vi "archive items in folder.vi"() -> ()   [LabVIEW 2009]
panel:
  in  "suffixes to remove":string[](array[string])=[".vi  ", ".llb", ".txt "]
  out "Errors":errorcluster[](array[cluster])
  # "doesn't remove suffixes"
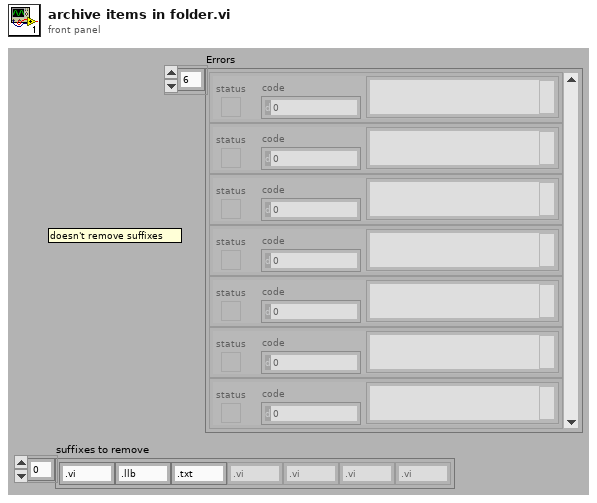
[diagram p1: front panel]
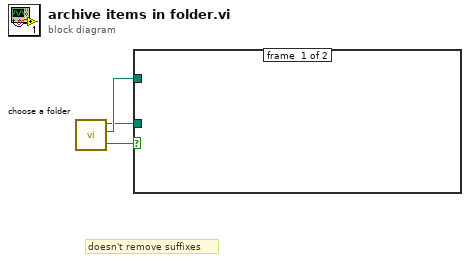
[diagram p0: block diagram]
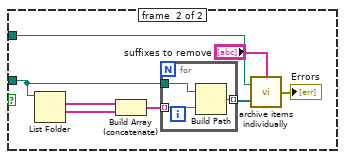
[diagram p2: hidden frame]
diagram:
  # "doesn't remove suffixes"
  n1 = call "choose a folder.vi"() -> ("OK"=w3:bool, "destination"=w2:path, "source"=w1:path)  [unwired: 4 in, 2 out]
  n2 = case shown="True" w3 {
    tunnel: w2 -> [_ w6]
    tunnel: w1 -> [_ w8]
    frame #0 {
    }
    frame #1 {
      n3 = List Folder(path=w8) -> (filenames=w11:string[], folder names=w10:string[])  [unwired: 3 in, 2 out]
      n4 = Build Array (concatenate)(w11, w10) -> (w9:string[])
      n5 = for {
        tunnel: w8 -> [w14]
        tunnel: w9 -> [w13] mode=indexing
        tunnel: [w12] -> w7 mode=indexing
        n6 = Build Path(base path=w14, name or relative path=w13) -> (appended path=w12:path)
      }
      n7 = call "archive items individually.vi"("suffixes to remove"="suffixes to remove", "Array 2"=w7, "destination folder"=w6) -> ("Errors"=→"Errors":errorcluster[])
    }
  }
